vi "Pulse - Set Trig DAQ Delay.vi"(8 "error in (no error)":errorcluster, 11 "3300 in":refnum<class "3300.lvclass">) -> (0 "error out":errorcluster, 3 "3300 out":refnum<class "3300.lvclass">)   [LabVIEW 2019, in "3300.lvlib" / "3300.lvclass"]
uses:
  Library/3300.lvclass
  Library/3300.lvclass/3300.ctl
  Accessors/Read Local Resource.vi
  Accessors/Write Local Resource.vi
  <instrlib>/Agilent N330X Series/Agilent N330X Series.lvlib
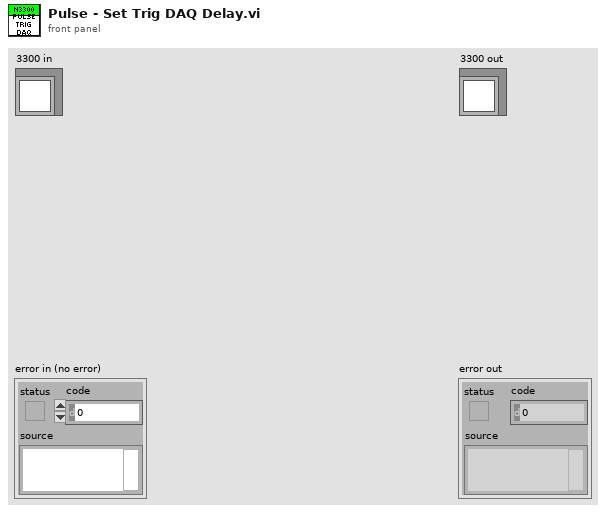
[diagram p1: front panel]
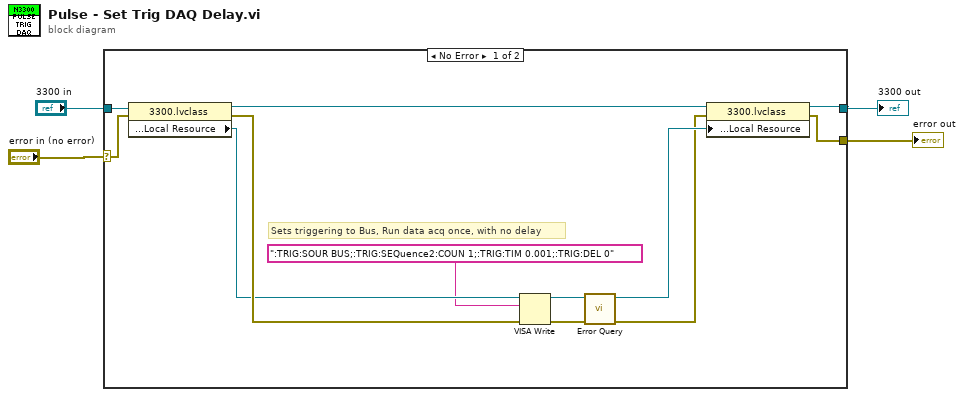
[diagram p0: block diagram]
diagram:
  n1 = case shown="No Error" "error in (no error)" {
    selector: "error in (no error)" -> [w14 w18]
    tunnel: [w8 w18] -> w1
    tunnel: [w12 w17] -> w2
    tunnel: "3300 in" -> [w6 w17]
    frame No Error {
      # "Sets triggering to Bus, Run data acq once, with no delay"
      n2 = property class="3300.lvclass"(reference=w6, error in=w14) -> (reference out=w11:refnum<class "3300.lvclass">, error out=w13:errorcluster, "Private:Accessors:Local Resource"=w7:refnum<visa-resource-name>)
      n3 = VISA Write(VISA resource name=w7, write buffer=":TRIG:SOUR BUS;:TRIG:SEQuence2:COUN 1;:TRIG:TIM 0.001;:TRIG:DEL 0" ("string (\"\")"), error in (no error)=w13) -> (VISA resource name out=w16:refnum<visa-resource-name>, error out=w15:errorcluster)  [unwired: 1 out]
      n4 = call <instrlib>:"Error Query.vi"("error in (no error)"=w15, "VISA resource name"=w16) -> ("error out"=w9:errorcluster, "VISA resource name out"=w10:refnum<visa-resource-name>)  [unwired: 6 in, 2 out]
      n5 = property class="3300.lvclass"(reference=w11, error in=w9, "Private:Accessors:Local Resource"=w10) -> (reference out=w12:refnum<class "3300.lvclass">, error out=w8:errorcluster)
    }
    frame Error {
    }
  }
  "error out" <- w1
  "3300 out" <- w2
